vi "Init_DSC.vi"(0 "Host_Reference":refnum<class "HGF_Reference.lvclass">, 2 "timeout in ms (-1)":i32=-1, 3 "Host Variable name":string, 5 "error in (no error)":errorcluster, 7 "Host Monitor timeout":i32=100, 9 "Agent Monitor timeout":i32=100) -> (10 "DSC Destination":refnum<class "HGF_TriggeredEvent.lvclass">, 12 "DSC Exception":refnum<class "HGF_TriggeredEvent.lvclass">, 13 "Host Monitor Trigger Event":refnum<class "HGF_Event.lvclass">, 14 "dup Host_Reference":refnum<class "HGF_Reference.lvclass">, 15 "Agent Monitor Trigger Event":refnum<class "HGF_Event.lvclass">, 16 "VarManagerEvent":refnum<class "HGF_Event.lvclass">, 17 "Host Variable":refnum<k21>, 18 "HGF_ThreadPool_Reference":refnum<class "HGF_Reference.lvclass">, 19 "error out":errorcluster)   [LabVIEW 2009, in "MoAgSy.lvlib" / "MoAgSy_Host.lvclass"]
doc: "Initializes Shared Variable Communication using DSC Module VIs\n-Creates Variable Manager\n-Creates Host-Variable\n-Creates DSC Monitor"
uses:
  MoAgSy_Host.lvclass
  HGF_BaseClasses/HGF_Reference/HGF_Reference.lvclass
  HGF_BaseClasses/HGF_Event/HGF_Event.lvclass
  HGF_BaseClasses/HGF_TriggeredEvent/HGF_TriggeredEvent.lvclass
  HGF_BaseClasses/HGF_Factory/HGF_Factory.lvclass
  HGF_BaseClasses/HGF_ThreadPool/HGF_ThreadPool.lvclass
  MoAgSy.lvlib
  HGF_DSC/HGF_DSCMonitor/HGF_DSCMonitor.lvclass
  HGF_DSC/HGF_DSCVarManager/HGF_DSCVarManager.lvclass
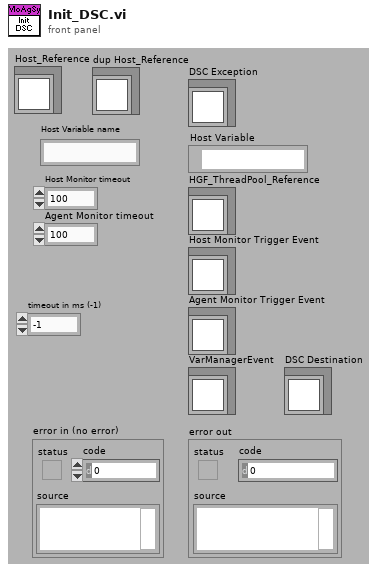
[diagram p1: front panel]
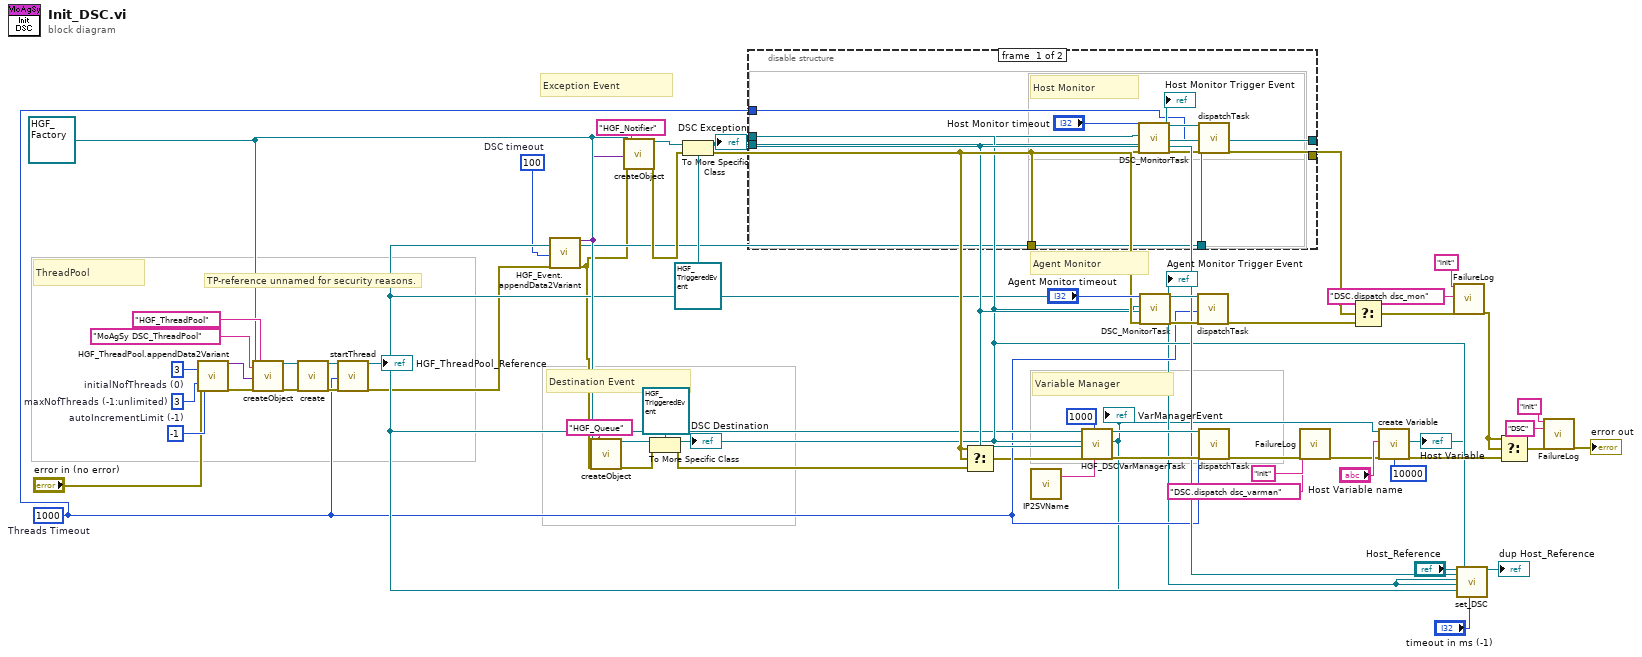
[diagram p0: block diagram]
diagram:
  w22 = 100  # DSC timeout
  w32 = refnum<class "HGF_Factory.lvclass"> refnum ("HGF_BaseClasses.lvlib:HGF_Factory.lvclass")
  w4 = 1000  # Threads Timeout
  w54 = 3  # initialNofThreads (0)
  w52 = 3  # maxNofThreads (-1:unlimited)
  w61 = -1  # autoIncrementLimit (-1)
  # "Destination Event"
  # "Exception Event"
  # "Agent Monitor"
  # "ThreadPool"
  # "TP-reference unnamed for security reasons."
  # "Variable Manager"
  n1 = call "HGF_ThreadPool.appendData2Variant.vi"("initialNofThreads (0)"=w54, "maxNofThreads (-1:unlimited)"=w52, "error in (no error)"="error in (no error)", "autoIncrementLimit (-1)"=w61) -> ("dup initData"=w55:variant, "error out"=w56:errorcluster)  [unwired: 3 in, 11 out]
  n2 = call "createObject.vi"("HGF_Factory"=w32, "objectName"="MoAgSy DSC_ThreadPool" ("string"), "initializationData"=w55, "error in (no error)"=w56, "className"="HGF_ThreadPool") -> ("HGF_Object"=w57:refnum<class "HGF_Factory.lvclass">, "error out"=w59:errorcluster)  [unwired: 13 out]
  n3 = call "create.vi"("Object"=w57, "error in (no error)"=w59) -> ("HGF_Reference"=w58:refnum<class "HGF_Reference.lvclass">, "error out"=w60:errorcluster)  [unwired: 1 in, 15 out]
  n4 = call "startThread.vi"("HGF_ThreadPool_Reference"=w58, "timeout in ms (-1)"=w4, "error in (no error)"=w60) -> ("dup HGF_ThreadPool_Reference"=w24:refnum<class "HGF_Reference.lvclass">, "error out"=w20:errorcluster)  [unwired: 15 out]
  "HGF_ThreadPool_Reference" <- w24
  n5 = call "HGF_Event.appendData2Variant.vi"("timeout in ms (-1)"=w22, "error in (no error)"=w20) -> ("dup initData"=w21:variant, "error out"=w19:errorcluster)  [unwired: 16 in]
  n6 = call "createObject.vi"("HGF_Factory"=w32, "initializationData"=w21, "error in (no error)"=w19, "className"="HGF_Queue") -> ("HGF_Object"=w34:refnum<class "HGF_Factory.lvclass">, "error out"=w35:errorcluster)  [unwired: 1 in, 13 out]
  n7 = call "createObject.vi"("HGF_Factory"=w32, "initializationData"=w21, "error in (no error)"=w19, "className"="HGF_Notifier") -> ("HGF_Object"=w45:refnum<class "HGF_Factory.lvclass">, "error out"=w42:errorcluster)  [unwired: 1 in, 13 out]
  n8 = To More Specific Class(target class=refnum<class "HGF_TriggeredEvent.lvclass"> refnum ("HGF_BaseClasses.lvlib:HGF_TriggeredEvent.lvclass"), reference=w34, error in=w35) -> (specific class reference=w26:refnum<class "HGF_TriggeredEvent.lvclass">, error out=w30:errorcluster)
  "DSC Destination" <- w26
  n9 = To More Specific Class(target class=refnum<class "HGF_TriggeredEvent.lvclass"> refnum ("HGF_BaseClasses.lvlib:HGF_TriggeredEvent.lvclass"), reference=w45, error in=w42) -> (specific class reference=w27:refnum<class "HGF_TriggeredEvent.lvclass">, error out=w31:errorcluster)
  "DSC Exception" <- w27
  n10 = disable-structure shown="Enabled" {
    disable-tunnel: [w70 _] -> w50
    disable-tunnel: w31 -> [w68 _]
    disable-tunnel: w27 -> [w67 _]
    disable-tunnel: w26 -> [w66 _]
    disable-tunnel: [w65 _] -> _
    disable-tunnel: w24 -> [w64 _]
    disable-tunnel: w4 -> [w63 _]
    frame #0 {
      # "Host Monitor"
      n11 = call "DSC_MonitorTask.vi"("Task Destination"=w66, "Task Exception Event"=w67, "error in (no error)"=w68, "timeout in ms (100)"="Host Monitor timeout") -> ("Monitor TaskLoop"=w72:refnum<class "HGF_TaskLoop.lvclass">, "Task Trigger Event"=w65:refnum<class "HGF_Event.lvclass">, "error out"=w71:errorcluster)  [unwired: 11 in, 2 out]
      "Host Monitor Trigger Event" <- w65
      n12 = call "dispatchTask.vi"("HGF_ThreadPool_Reference"=w64, "HGF_ThreadTask"=w72, "timeout in ms (-1)"=w63, "error in (no error)"=w71) -> ("error out"=w70:errorcluster)  [unwired: 13 in, 2 out]
    }
    frame #1 {
    }
  }
  n13 = Select(t=w31, s=w31, f=w30) -> (s? t:f=w2:errorcluster)
  n14 = call "IP2SVName.vi"() -> ("name"=w37:string)  [unwired: 19 in]
  n15 = call "HGF_DSCVarManagerTask.vi"("Task Destination"=w26, "Task Exception Event"=w27, "error in (no error)"=w2, "timeout in ms (10000)"=1000, "object/ProcessName"=w37) -> ("VarManager TaskLoop"=w40:refnum<class "HGF_TaskLoop.lvclass">, "Task Trigger Event"=w1:refnum<class "HGF_Event.lvclass">, "error out"=w39:errorcluster)  [unwired: 10 in, 2 out]
  "VarManagerEvent" <- w1
  n16 = call "DSC_MonitorTask.vi"("Task Destination"=w26, "Task Exception Event"=w27, "error in (no error)"=w31, "timeout in ms (100)"="Agent Monitor timeout") -> ("Monitor TaskLoop"=w47:refnum<class "HGF_TaskLoop.lvclass">, "Task Trigger Event"=w3:refnum<class "HGF_Event.lvclass">, "error out"=w49:errorcluster)  [unwired: 11 in, 2 out]
  "Agent Monitor Trigger Event" <- w3
  n17 = call "dispatchTask.vi"("HGF_ThreadPool_Reference"=w24, "HGF_ThreadTask"=w47, "timeout in ms (-1)"=w4, "error in (no error)"=w49) -> ("error out"=w48:errorcluster)  [unwired: 13 in, 2 out]
  n18 = call "dispatchTask.vi"("HGF_ThreadPool_Reference"=w24, "HGF_ThreadTask"=w40, "timeout in ms (-1)"=w4, "error in (no error)"=w39) -> ("error out"=w13:errorcluster)  [unwired: 13 in, 2 out]
  n19 = call "FailureLog.vi"("Section"="init", "key"="DSC.dispatch dsc_varman", "error in (no error)"=w13) -> ("error out"=w12:errorcluster)  [unwired: 16 in]
  n20 = Select(t=w50, s=w50, f=w48) -> (s? t:f=w17:errorcluster)
  n21 = call "create Variable.vi"("Variable Manager Trigger Event"=w1, "Variable name"="Host Variable name", "timeout"=10000, "error in (no error)"=w12) -> ("Variable"=w25:refnum<k21>, "error out"=w38:errorcluster)  [unwired: 13 in, 1 out]
  "Host Variable" <- w25
  n22 = call "FailureLog.vi"("Section"="init", "key"="DSC.dispatch dsc_mon", "error in (no error)"=w17) -> ("error out"=w16:errorcluster)  [unwired: 16 in]
  n23 = call "set_DSC.vi"("Host_Reference"="Host_Reference", "DSCException"=w27, "Host_Event"=w3, "Agent_Event"=w3, "ManagerEvent"=w1, "DSCDestination"=w26, "Host Variable"=w25, "timeout in ms (-1)"="timeout in ms (-1)", "MoAgSy_DSCThreadPool"=w24) -> ("dup Host_Reference"=→"dup Host_Reference":refnum<class "HGF_Reference.lvclass">)  [unwired: 9 in, 1 out]
  n24 = Select(t=w16, s=w16, f=w38) -> (s? t:f=w9:errorcluster)
  n25 = call "FailureLog.vi"("Section"="init", "key"="DSC", "error in (no error)"=w9) -> ("error out"=→"error out":errorcluster)  [unwired: 16 in]
